vi "synnax writer open Array.vi"(4 "enable_auto_commit (T)":bool=TRUE, 5 "err_on_unauthorized (F)":bool, 6 "auto_index (F)":bool, 7 "start (now)":timestamp, 8 "error in":errorcluster, 9 "authorities (255 for all channels)":u8[](array[numeric]), 10 "channels in":u32[](array[numeric]), 11 "client in":u64) -> (0 "error out":errorcluster, 2 "channels out":u32[](array[numeric]), 3 "writer out":u64)   [LabVIEW 2026, in "synnax_clib.lvlib"]
doc: "SYNNAX_EXPORT int32_t synnax_writer_open(\n SynnaxClient client,\n int64_t start,\n const uint32_t *channels,\n uint64_t channel_count,\n int32_t mode,\n int32_t enable_auto_commit,\n SynnaxWriter *out_writer,\n SynnaxError err\n);"
uses:
  typedefs/writer_mode.ctl
  Timestamp Conversion Single.vi
  synnax_clib.lvlib
  synnax_clib.dll
panel:
  out "client out":u64
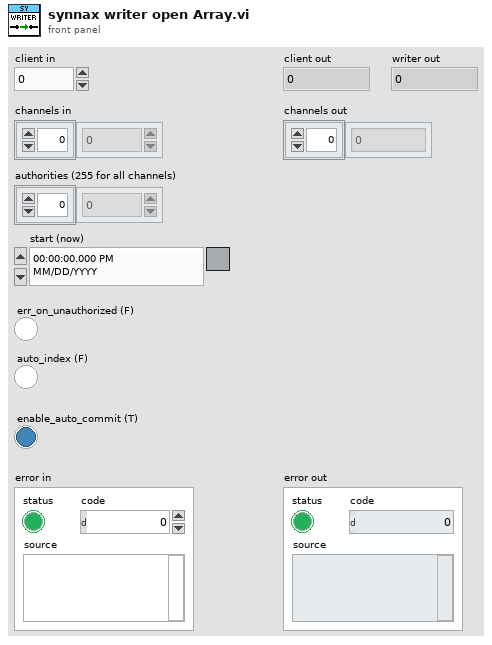
[diagram p1: front panel]
types:
  T1 = typedef "synnax_clib.lvlib/writer_mode.ctl" = enum16{"PERSIST & STREAM", "PERSIST", "STREAM"}
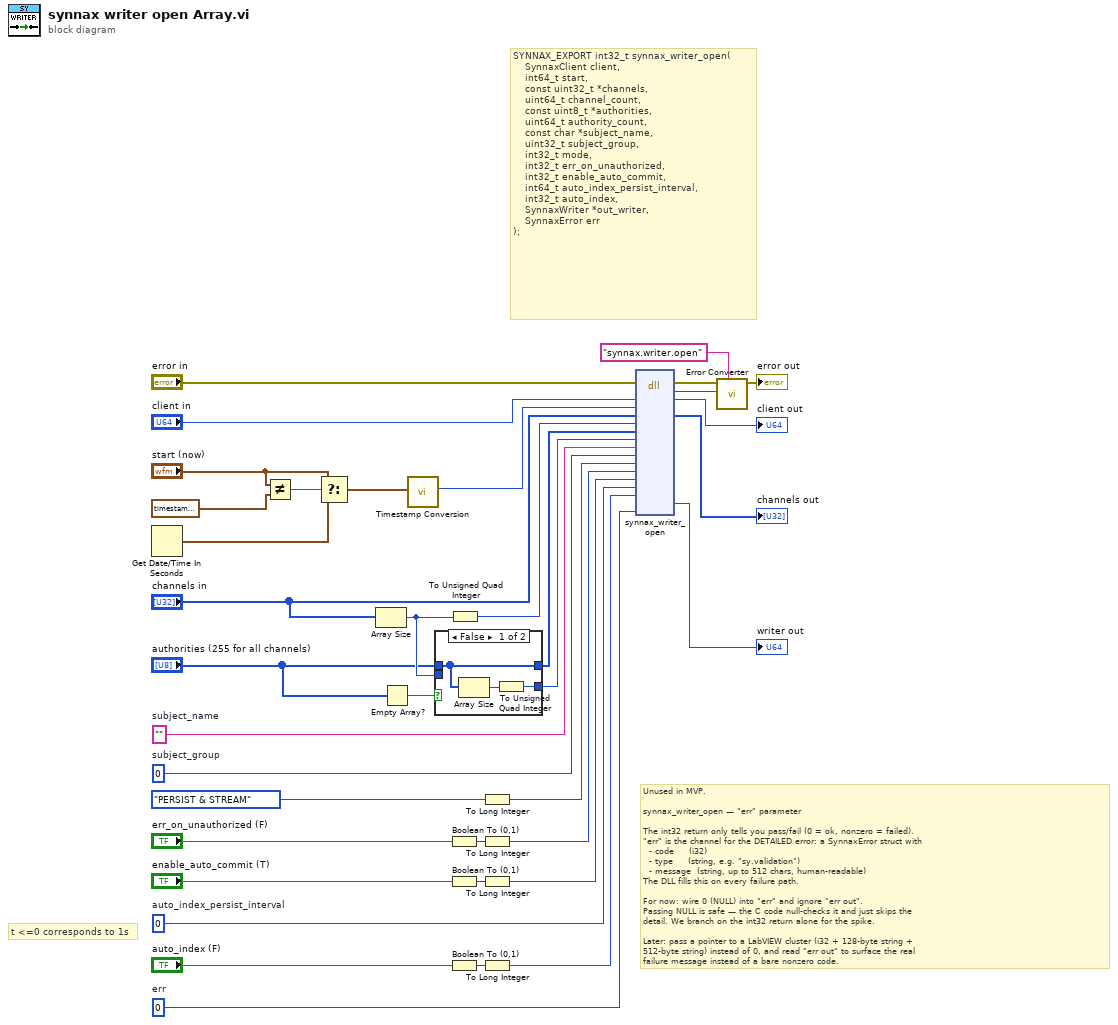
[diagram p0: block diagram]
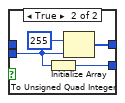
[diagram p2: hidden frame]
diagram:
  w17 = i64 0  # auto_index_persist_interval
  w21 = u32 0  # subject_group
  w22 = ""  # subject_name
  w32 = u64 0  # err
  # "t <=0 corresponds to 1s"
  # "Unused in MVP.\n\nsynnax_writer_open — \"err\" parameter\n\nThe int32 return only tells you pass/fail (0 = ok, nonzero = failed).\n\"err\" is the channel for the DETAILED error: a SynnaxError struct with\n  - code     (i32)\n  - type     (string, e.g. \"sy.validation\")\n  - message  (string, up to 512 chars, human-readable)\nThe DLL fills this on every failure path.\n\nFor now: wire 0 (NULL) into \"err\" and ignore \"err out\".\nPassing NULL is safe — the C code null-checks it and just skips the\ndetail. We branch on the int32 return alone for the spike.\n\nLater: pass a pointer to a LabVIEW cluster (i32 + 128-byte string +\n512-byte string) instead of 0, and read \"err out\" to surface the real\nfailure message instead of a bare nonzero code."
  # "SYNNAX_EXPORT int32_t synnax_writer_open(\n    SynnaxClient client,\n    int64_t start,\n    const uint32_t *channels,\n    uint64_t channel_count,\n    const uint8_t *authorities,\n    uint64_t authority_count,\n    const char *subject_name,\n    uint32_t subject_group,\n    int32_t mode,\n    int32_t err_on_unauthorized,\n    int32_t enable_auto_commit,\n    int64_t auto_index_persist_interval,\n    int32_t auto_index,\n    SynnaxWriter *out_writer,\n    SynnaxError err\n);"
  n1 = Get Date/Time In Seconds() -> (seconds since 1Jan1904=w4:timestamp)
  n2 = Not Equal?(x="start (now)", y=timestamp timestamp(0 s since 1904-01-01)) -> (x != y?=w7:bool)
  n3 = Select(t="start (now)", s=w7, f=w4) -> (s? t:f=w3:timestamp)
  n4 = Array Size(array="channels in") -> (size(s)=w12:i32)
  n5 = Empty Array?(array="authorities (255 for all channels)") -> (empty?=w10:bool)
  n6 = call-poly "Timestamp Conversion.vi"("timestamp"=w3) -> ("timestamp (ns)"=w2:i64)  [unwired: 9 in]
  n7 = case shown="False" w10 {
    tunnel: [w39 w44] -> w13
    tunnel: w12 -> [_ w42]
    tunnel: "authorities (255 for all channels)" -> [w39 _]
    tunnel: [w38 w41] -> w8
    frame False {
      n8 = Array Size(array=w39) -> (size(s)=w40:i32)
      n9 = To Unsigned Quad Integer(1:w40) -> (0:w38:u64)
    }
    frame True {
      n10 = To Unsigned Quad Integer(1:w42) -> (0:w41:u64)
      n11 = Initialize Array(u8 255, w42) -> (w44:u8[])
    }
  }
  n12 = Boolean To (0,1)(Boolean="err_on_unauthorized (F)") -> (0, 1=w19:i16)
  n13 = Boolean To (0,1)(Boolean="enable_auto_commit (T)") -> (0, 1=w33:i16)
  n14 = Boolean To (0,1)(Boolean="auto_index (F)") -> (0, 1=w15:i16)
  n15 = To Unsigned Quad Integer(1:w12) -> (0:w11:u64)
  n16 = To Long Integer(number=writer_mode."PERSIST & STREAM") -> (32bit integer=w23:i32)
  n17 = To Long Integer(number=w19) -> (32bit integer=w18:i32)
  n18 = To Long Integer(number=w33) -> (32bit integer=w31:i32)
  n19 = To Long Integer(number=w15) -> (32bit integer=w14:i32)
  n20 = dll-call lib="C/synnax/client/labview/synnax_clib.*" fn="synnax_writer_open"(error in="error in", "client"="client in", "start"=w2, "channels"="channels in", "channel_count"=w11, "authorities"=w13, "authority_count"=w8, "subject_name"=w22, "subject_group"=w21, "mode"=w23, "err_on_unauthorized"=w18, "enable_auto_commit"=w31, "auto_index_persist_interval"=w17, "auto_index"=w14, "err"=w32) -> (error out=w30:errorcluster, "return type"=w29:i32, "client"=→"client out":u64, "channels"=→"channels out":u32[], "out_writer"=→"writer out":u64)  [unwired: 15 in, 1 out]
  n21 = call "Error Converter.vi"("source"="synnax.writer.open", "error code"=w29, "error in (no error)"=w30) -> ("error out"=→"error out":errorcluster)  [unwired: 8 in]
